vi "Circus Critical PCs List.vi"(6 "Init":bool, 8 "error in (no error)":errorcluster) -> (0 "error out":errorcluster, 3 "Critical PC List out":string[](array[string]))   [LabVIEW 2026, in "TALOS.lvlib"]
doc: "This VI contains the list of all the AEgIS PCs names (machine names)."
uses:
  TALOS.lvlib
  Ancestor/Ancestor/Ancestor.lvclass/Ancestor.ctl
  Generate Error.vi
  Circus Root Path.vi
  TALOS Config Param.vi
  FGV/Error Memory/Get Error Description.vi
  Get PC name.vi
  Ancestor/Ancestor/Read ID.vi
  Get Class Name.vi
  <vilib>/Utility/error.llb/Clear Errors.vi
  FGV/Error Memory/Error Memory Core.vi
  <vilib>/AdvancedString/Delimited String to 1D String Array.vi
  <vilib>/AdvancedString/Delimited String to 1D String Array (string).vi
  FGV/Error Memory/Error Crt Lvl checker.vi
  FGV/Error Memory/Error Memory Core.vi/40c8088d-b597-4017-91af-faa98e00292e.vi
  FGV/Error Memory/Error Memory Core.vi/d4a3ab98-063c-4e44-b43d-fbdcfe6c2be2.vi
  Global Memory.vi
  Global Constants.vi
  <vilib>/Utility/LVClass/Get LV Class Name.vi
  Is in Packed Library.vi
  TALOS Root path.vi
  Read CSV worksheet.vi
  <vilib>/Utility/error.llb/General Error Handler.vi
  <vilib>/Utility/config.llb/Open Config Data.vi
  <vilib>/Utility/config.llb/Get Section Names.vi
  <vilib>/Utility/config.llb/Get Key Names.vi
  <vilib>/Utility/config.llb/Read Key.vi
  <vilib>/Utility/config.llb/Read Key (String).vi
  <vilib>/Utility/config.llb/Close Config Data.vi
  Ancestor/Ancestor/Ancestor.lvclass
  <vilib>/Comparison/Equal/Equal Functor/Equal Functor.lvclass
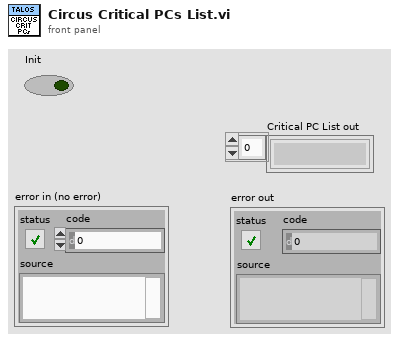
[diagram p1: front panel]
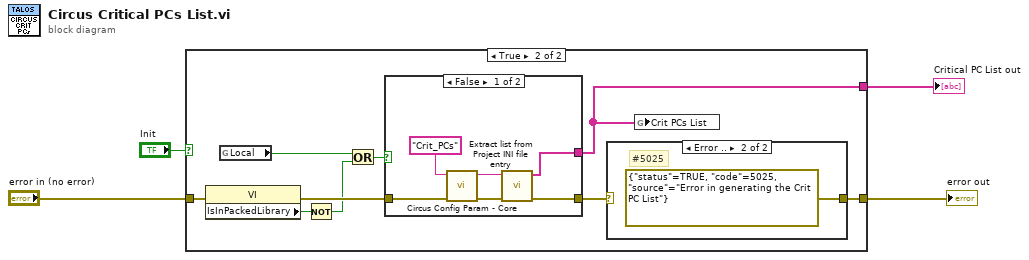
[diagram p0: block diagram]
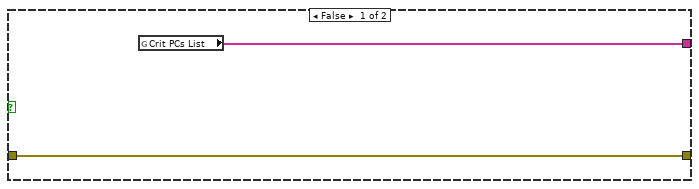
[diagram p2: hidden frame]
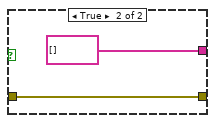
[diagram p3: hidden frame]
diagram:
  n1 = case shown="True" "Init" {
    tunnel: [w5 w9] -> w2
    tunnel: "error in (no error)" -> [w6 w15]
    tunnel: [w6 w7] -> w4
    frame False {
      n2 = global read "Global Memory.vi" "Crit PCs List"() -> (w5:string[])
    }
    frame True {
      n3 = property class="VI"(error in=w15) -> (error out=w14:errorcluster, "IsInPackedLibrary"=w12:bool)  [unwired: 1 in, 1 out]
      n4 = global read "Global Constants.vi" "Local"() -> (w10:bool)
      n5 = Not(x=w12) -> (.not. x?=w11:bool)
      n6 = Or(x=w10, y=w11) -> (x .or. y?=w13:bool)
      n7 = case shown="False" w13 {
        tunnel: [w16 string[] []] -> w9
        tunnel: w14 -> [w20 w23]
        tunnel: [w18 w23] -> w8
        frame False {
          n8 = call "Circus Config Param - Core.vi"("error in (no error)"=w20, "Parameter Name"="Crit_PCs") -> ("error out"=w19:errorcluster, "Output"=w17:string)  [unwired: 8 in]
          n9 = call "Extract list from Project INI file entry.vi"("error in (no error)"=w19, "Entry from INI file"=w17) -> ("error out"=w18:errorcluster, "Array"=w16:string[])  [unwired: 8 in]
        }
        frame True {
        }
      }
      n10 = case shown="Error .." w8 {
        selector: w8 -> [w24 _]
        tunnel: [w24 errorcluster {"status"=TRUE, "code"=5025, "source"="Error in generating the Crit PC List"} ("error IO")] -> w7
        frame No Error {
        }
        frame Error {
          # "#5025"
        }
      }
      n11 = global write "Global Memory.vi" "Crit PCs List"(w9) -> ()
    }
  }
  "Critical PC List out" <- w2
  "error out" <- w4
